vi "CameraStreamAttribute.vi"() -> ()   [LabVIEW 2022 SP3]
uses:
  <vilib>/userdefined/High Color/IMAQdx.ctl
  <vilib>/vision/driver/NI_Vision_Acquisition_Software.lvlib
  <resource>/objmgr/imaqdx.rc
panel:
  in  "Session In":T1
  out "Image":T2(plugin-control)
  in  "Stop":bool
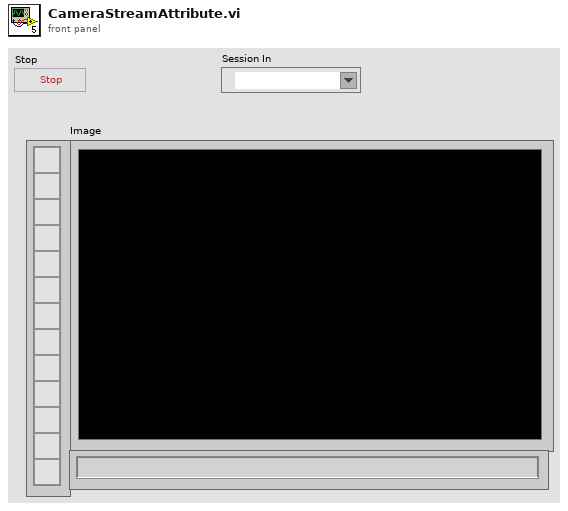
[diagram p1: front panel]
types:
  T1 = typedef "IMAQdx.ctl" = refnum<k21>
  T2 = typedef "IMAQ Image.ctl" = refnum<image>
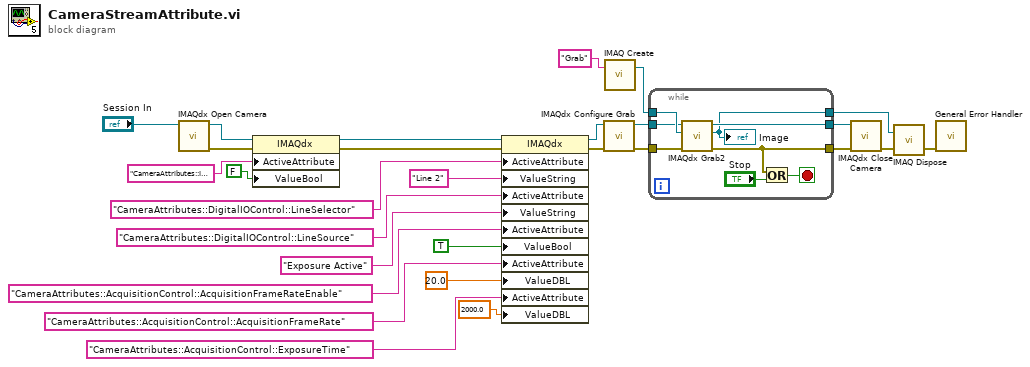
[diagram p0: block diagram]
diagram:
  n1 = call <vilib>:"IMAQdx Open Camera.vi"("Session In"="Session In") -> ("error out"=w17:errorcluster, "Session Out"=w18:T1)  [unwired: 9 in]
  n2 = property class="IMAQdx"(reference=w18, error in=w17, "ActiveAttribute"="CameraAttributes::ImageFormatControl::ReverseX", "ValueBool"=FALSE) -> (reference out=w7:T1, error out=w5:errorcluster)
  n3 = property class="IMAQdx"(reference=w7, error in=w5, "ActiveAttribute"="CameraAttributes::DigitalIOControl::LineSelector", "ValueString"="Line 2", "ActiveAttribute"="CameraAttributes::DigitalIOControl::LineSource", "ValueString"="Exposure Active", "ActiveAttribute"="CameraAttributes::AcquisitionControl::AcquisitionFrameRateEnable", "ValueBool"=TRUE, "ActiveAttribute"="CameraAttributes::AcquisitionControl::AcquisitionFrameRate", "ValueDBL"=20.0, "ActiveAttribute"="CameraAttributes::AcquisitionControl::ExposureTime", "ValueDBL"=2000.0) -> (reference out=w6:T1, error out=w4:errorcluster)
  n4 = call <vilib>:"IMAQdx Configure Grab.vi"("error in"=w4, "Session In"=w6) -> ("error out"=w19:errorcluster, "Session Out"=w20:T1)  [unwired: 8 in]
  n5 = call "IMAQ Create"("Image Name"="Grab") -> ("New Image"=w27:T2)  [unwired: 4 in, 1 out]
  n6 = while {
    tunnel: w19 -> [w31]
    tunnel: w27 -> [w34]
    tunnel: w20 -> [w33]
    tunnel: [w30] -> w25
    tunnel: [w29] -> w26
    tunnel: [w32] -> w24
    stop <- w35 stop-if-true
    n7 = call <vilib>:"IMAQdx Grab2.vi"("error in"=w31, "Image In"=w34, "Session In"=w33) -> ("error out"=w30:errorcluster, "Image Out"=w29:T2, "Session Out"=w32:T1)  [unwired: 5 in, 1 out]
    "Image" <- w29
    n8 = Or(x=w30, y="Stop") -> (x .or. y?=w35:bool)
  }
  n9 = call <vilib>:"IMAQdx Close Camera.vi"("error in"=w25, "Session In"=w24) -> ("error out"=w23:errorcluster)  [unwired: 9 in]
  n10 = call "IMAQ Dispose"("Image"=w26, "error in (no error)"=w23) -> ("error out"=w22:errorcluster)  [unwired: 4 in]
  n11 = call <vilib>:"General Error Handler.vi"("error in (no error)"=w22) -> ()  [unwired: 10 in, 5 out]
